vi "Three part faster.vi"() -> ()   [LabVIEW 2009]
uses:
  <vilib>/vision/Image Controls.llb/IMAQ Image.ctl
  <vilib>/Analysis/3filter.llb/Filter Passband Type.ctl
  <vilib>/Analysis/3filter.llb/Butterworth Filter (DBL).vi
  <vilib>/Instr/_visa.llb/VISA Configure Serial Port (Instr).vi
  <vilib>/vision/NI_Vision_Development_Module.lvlib
  <vilib>/Analysis/NI_AALBase.lvlib
panel:
  out "decimal integer string 2":string
  out "number 2":u32
  out "cluster 2":T1
  in  "Orange Guitar":T2={"Global Rectangle"=[587, 282, 628, 378], "Contours"=[{"ID"=enum."External", "Type"=2, "Coordinates"=[627, 377, 587, 282]}]} {"Contours"."Type" items=["No Selection", "Point", "Line", "Rectangle", "Oval", "Polygon", "Freehand Region", "Annulus", "Unused2", "Unused3", "Broken Line", "Freehand Line", "Rotated Rectangle"]}
  in  "Yellow Guitar":T2={"Global Rectangle"=[546, 282, 563, 376], "Contours"=[{"ID"=enum."External", "Type"=2, "Coordinates"=[562, 375, 546, 282]}]} {"Contours"."Type" items=["No Selection", "Point", "Line", "Rectangle", "Oval", "Polygon", "Freehand Region", "Annulus", "Unused2", "Unused3", "Broken Line", "Freehand Line", "Rotated Rectangle"]}
  in  "Green Guitar":T2={"Global Rectangle"=[498, 284, 505, 376], "Contours"=[{"ID"=enum."External", "Type"=2, "Coordinates"=[498, 375, 504, 284]}]} {"Contours"."Type" items=["No Selection", "Point", "Line", "Rectangle", "Oval", "Polygon", "Freehand Region", "Annulus", "Unused2", "Unused3", "Broken Line", "Freehand Line", "Rotated Rectangle"]}
  in  "Blue Guitar":T2={"Global Rectangle"=[569, 290, 594, 372], "Contours"=[{"ID"=enum."External", "Type"=2, "Coordinates"=[593, 371, 569, 290]}]} {"Contours"."Type" items=["No Selection", "Point", "Line", "Rectangle", "Oval", "Polygon", "Freehand Region", "Annulus", "Unused2", "Unused3", "Broken Line", "Freehand Line", "Rotated Rectangle"]}
  in  "Red Guitar":T2={"Global Rectangle"=[526, 284, 530, 370], "Contours"=[{"ID"=enum."External", "Type"=2, "Coordinates"=[529, 369, 526, 284]}]} {"Contours"."Type" items=["No Selection", "Point", "Line", "Rectangle", "Oval", "Polygon", "Freehand Region", "Annulus", "Unused2", "Unused3", "Broken Line", "Freehand Line", "Rotated Rectangle"]}
  out "Blue Guitar":dbl[](graph)
  out "Yellow Guitar":dbl[](graph)
  out "Yellow Guitar LED":bool
  out "Green Guitar":dbl[](graph)
  out "Green Guitar LED":bool
  out "Red Guitar":dbl[](graph)
  out "Red Guitar LED":bool
  out "Blue Guitar LED":bool
  out "Orange Guitar":dbl[](graph)
  out "Orange Guitar LED":bool
  in  "Orange Bass":T2={"Global Rectangle"=[220, 296, 225, 371], "Contours"=[{"ID"=enum."External", "Type"=2, "Coordinates"=[224, 370, 220, 296]}]} {"Contours"."Type" items=["No Selection", "Point", "Line", "Rectangle", "Oval", "Polygon", "Freehand Region", "Annulus", "Unused2", "Unused3", "Broken Line", "Freehand Line", "Rotated Rectangle"]}
  out "Orange Bass":dbl[](graph)
  out "Orange Bass LED":bool
  in  "Green Bass":T2={"Global Rectangle"=[100, 292, 131, 371], "Contours"=[{"ID"=enum."External", "Type"=2, "Coordinates"=[100, 370, 130, 292]}]} {"Contours"."Type" items=["No Selection", "Point", "Line", "Rectangle", "Oval", "Polygon", "Freehand Region", "Annulus", "Unused2", "Unused3", "Broken Line", "Freehand Line", "Rotated Rectangle"]}
  in  "Blue Bass":T2={"Global Rectangle"=[193, 293, 199, 374], "Contours"=[{"ID"=enum."External", "Type"=2, "Coordinates"=[193, 373, 198, 293]}]} {"Contours"."Type" items=["No Selection", "Point", "Line", "Rectangle", "Oval", "Polygon", "Freehand Region", "Annulus", "Unused2", "Unused3", "Broken Line", "Freehand Line", "Rotated Rectangle"]}
  in  "Red Bass":T2={"Global Rectangle"=[129, 294, 154, 376], "Contours"=[{"ID"=enum."External", "Type"=2, "Coordinates"=[129, 375, 153, 294]}]} {"Contours"."Type" items=["No Selection", "Point", "Line", "Rectangle", "Oval", "Polygon", "Freehand Region", "Annulus", "Unused2", "Unused3", "Broken Line", "Freehand Line", "Rotated Rectangle"]}
  in  "Yellow Bass":T2={"Global Rectangle"=[160, 295, 175, 378], "Contours"=[{"ID"=enum."External", "Type"=2, "Coordinates"=[160, 377, 174, 295]}]} {"Contours"."Type" items=["No Selection", "Point", "Line", "Rectangle", "Oval", "Polygon", "Freehand Region", "Annulus", "Unused2", "Unused3", "Broken Line", "Freehand Line", "Rotated Rectangle"]}
  out "Blue Bass":dbl[](graph)
  out "Yellow Bass":dbl[](graph)
  out "Yellow Bass LED":bool
  out "Green Bass":dbl[](graph)
  out "Green Bass LED":bool
  out "Red Bass":dbl[](graph)
  out "Red Bass LED":bool
  out "Blue Bass LED":bool
  in  "Mask":T2 {"Contours"."Type" items=["No Selection", "Point", "Line", "Rectangle", "Oval", "Polygon", "Freehand Region", "Annulus", "Unused2", "Unused3", "Broken Line", "Freehand Line", "Rotated Rectangle"]}
  in  "Red Line":T2={"Global Rectangle"=[300, 297, 320, 380], "Contours"=[{"ID"=enum."External", "Type"=2, "Coordinates"=[300, 379, 319, 297]}]} {"Contours"."Type" items=["No Selection", "Point", "Line", "Rectangle", "Oval", "Polygon", "Freehand Region", "Annulus", "Unused2", "Unused3", "Broken Line", "Freehand Line", "Rotated Rectangle"]}
  out "Waveform Red":dbl[](graph)
  out "LED Red":bool
  in  "Blue Line":T2={"Global Rectangle"=[374, 278, 383, 377], "Contours"=[{"ID"=enum."External", "Type"=2, "Coordinates"=[382, 376, 374, 278]}]} {"Contours"."Type" items=["No Selection", "Point", "Line", "Rectangle", "Oval", "Polygon", "Freehand Region", "Annulus", "Unused2", "Unused3", "Broken Line", "Freehand Line", "Rotated Rectangle"]}
  in  "Green Line":T2={"Global Rectangle"=[406, 309, 423, 383], "Contours"=[{"ID"=enum."External", "Type"=2, "Coordinates"=[422, 382, 406, 309]}]} {"Contours"."Type" items=["No Selection", "Point", "Line", "Rectangle", "Oval", "Polygon", "Freehand Region", "Annulus", "Unused2", "Unused3", "Broken Line", "Freehand Line", "Rotated Rectangle"]}
  out "Waveform Green":dbl[](graph)
  out "LED Green":bool
  in  "Yellow Line":T2={"Global Rectangle"=[342, 292, 349, 377], "Contours"=[{"ID"=enum."External", "Type"=2, "Coordinates"=[342, 376, 348, 292]}]} {"Contours"."Type" items=["No Selection", "Point", "Line", "Rectangle", "Oval", "Polygon", "Freehand Region", "Annulus", "Unused2", "Unused3", "Broken Line", "Freehand Line", "Rotated Rectangle"]}
  out "cluster":T1
  in  "baud rate (9600)":u32=9600
  in  "VISA resource name":refnum<visa-resource-name>
  out "number":u32
  out "decimal integer string":string
  out "Image Dst Out":T3
  out "LED Yellow":bool
  out "Waveform Yellow":dbl[](graph)
  in  "playtime":dbl=30.0
  out "Frame Number":i32
  in  "Frame Start":i32=2400
  out "Blue Drum":bool
  out "Blue Drum":dbl[](graph)
  in  "stop":bool
  in  "AVI Path":path
  # "BLUE"
  # "YELLOW"
  # "GREEN"
  # "RED"
  # "Drums"
  # "Bass"
  # "Guitar"
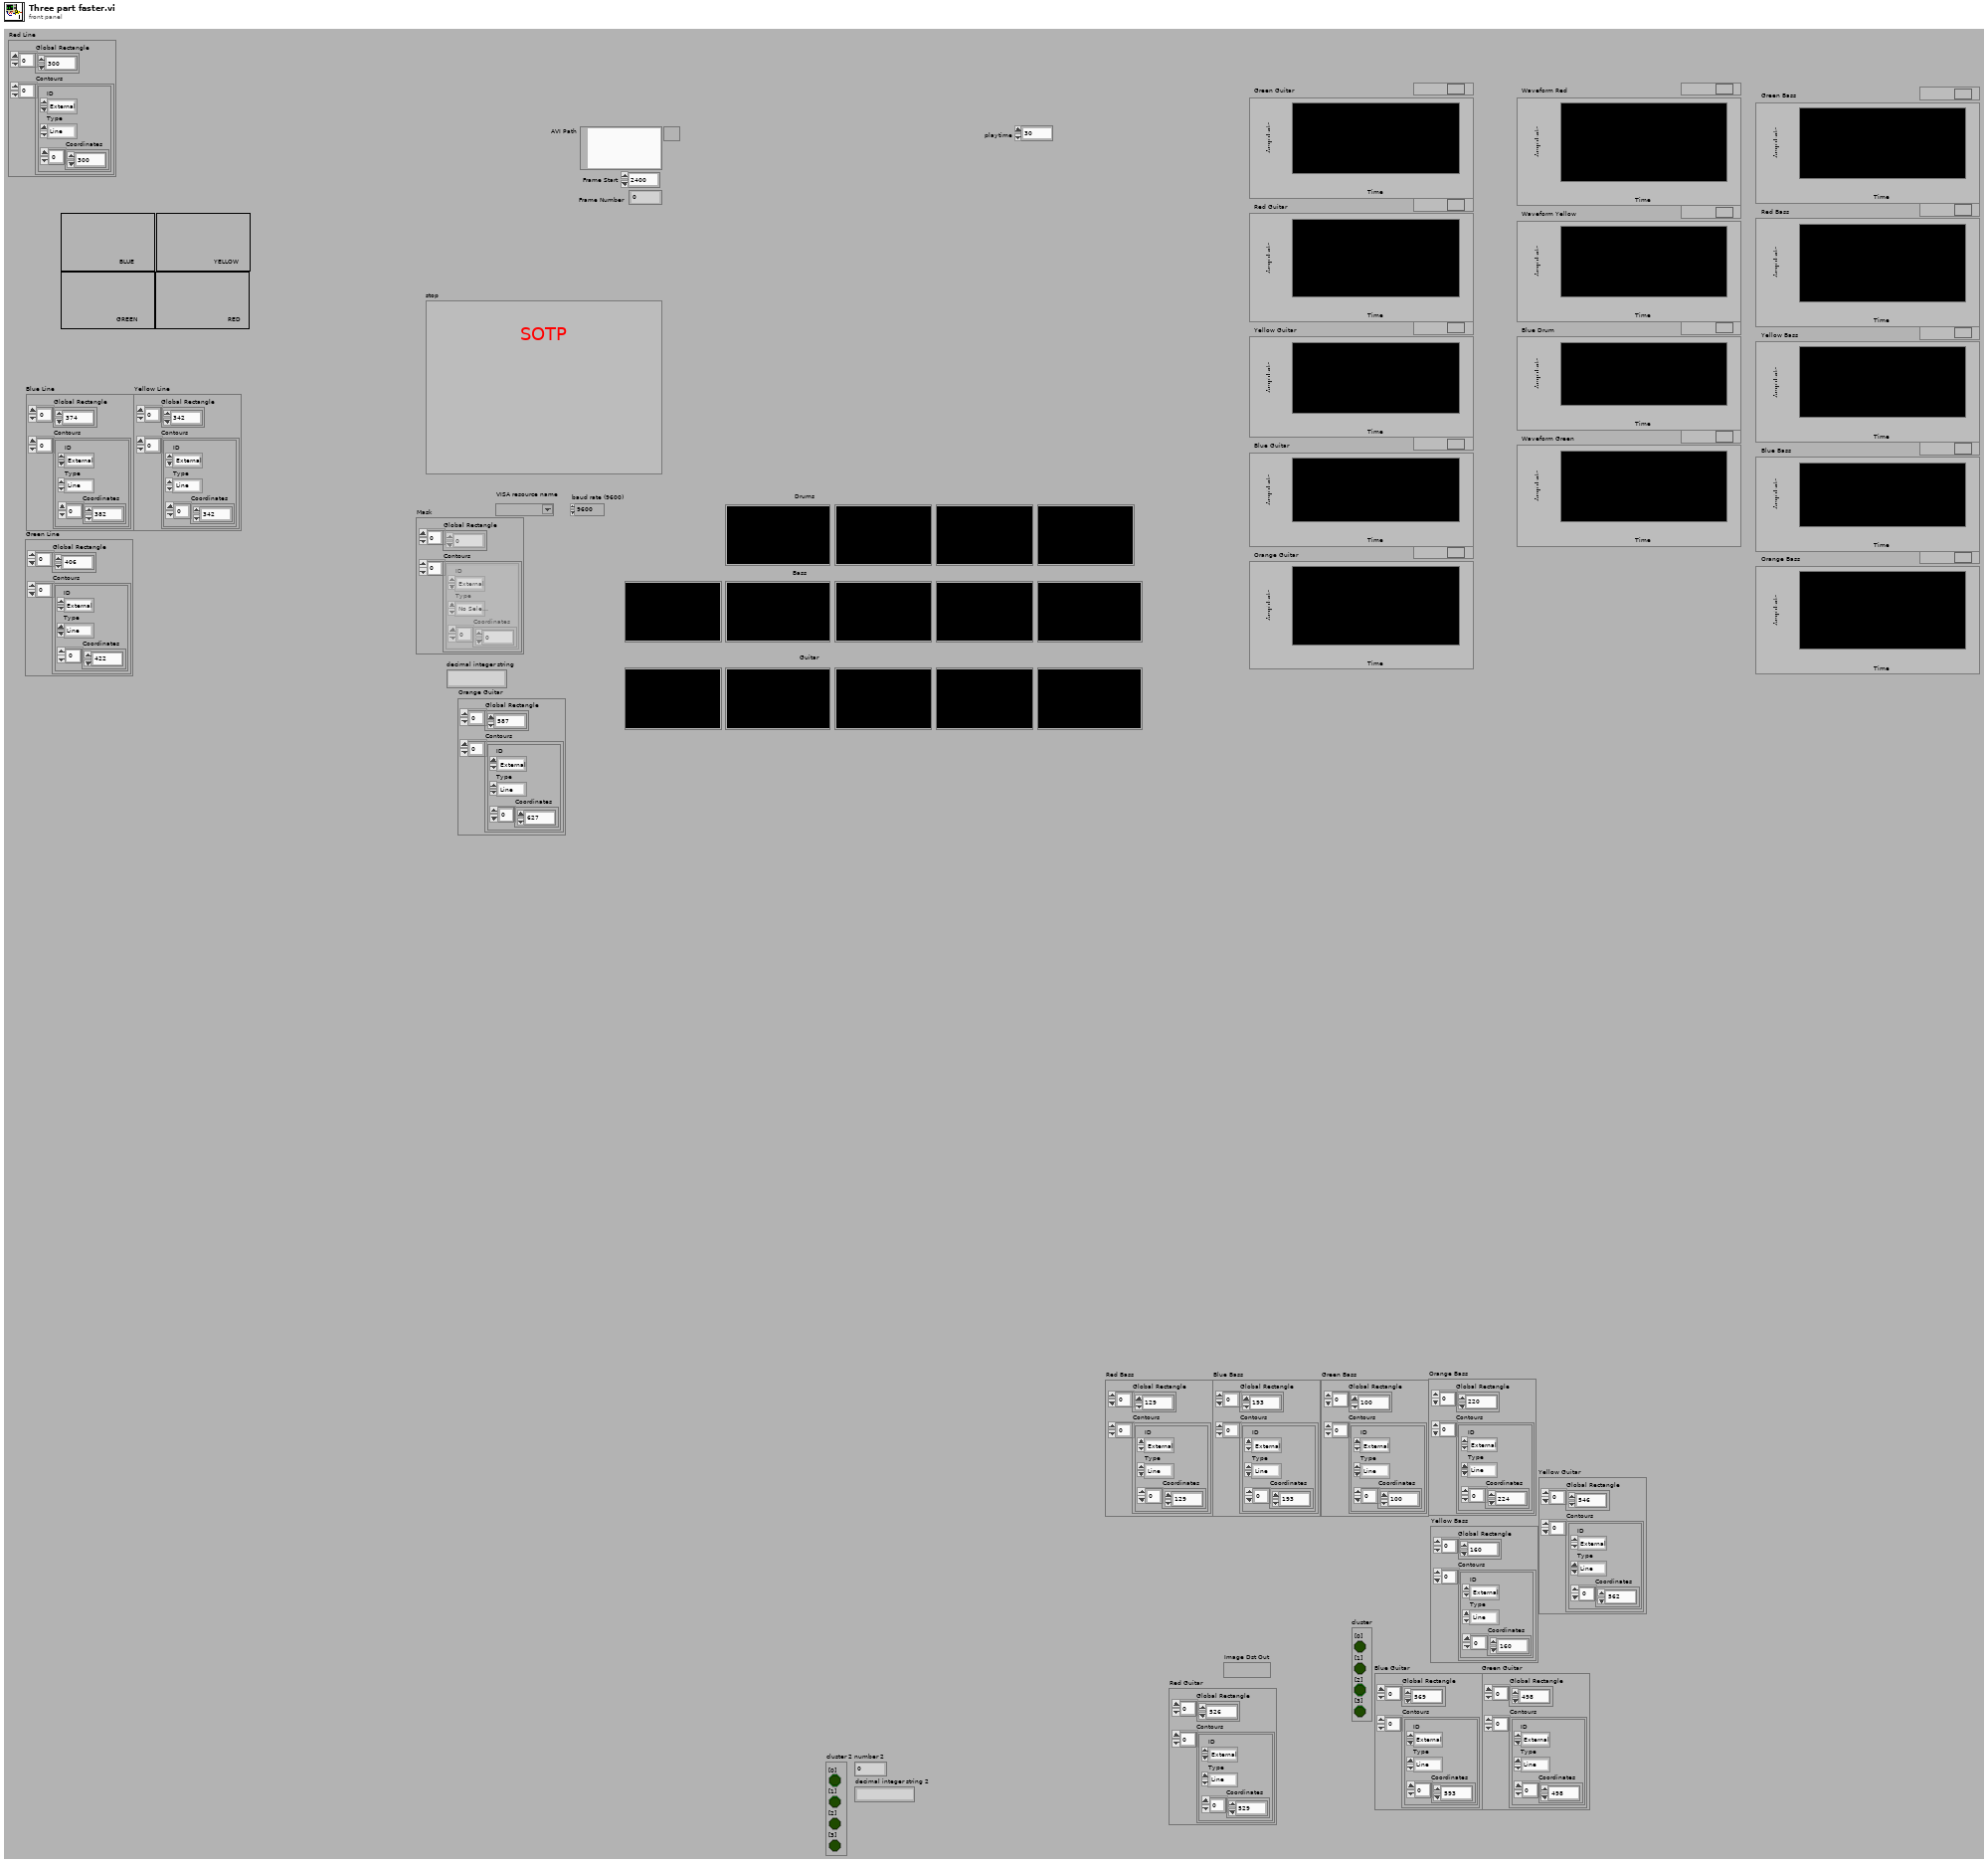
[diagram p1: front panel]
types:
  T1 = cluster{"[0]":bool, "[1]":bool, "[2]":bool, "[3]":bool, "[4]":bool, "[5]":bool, "[6]":bool, "[7]":bool, "[8]":bool}
  T2 = cluster{"Global Rectangle":i32[], "Contours":cluster{"ID":enum32{"External", "Internal"}, "Type":u32, "Coordinates":i32[]}[]}
  T3 = typedef "IMAQ Image.ctl" = refnum<image>
  T4 = typedef "NI_AALBase.lvlib/Filter Passband Type.ctl" = enum32{"Lowpass", "Highpass", "Bandpass", "Bandstop"}
  T5 = typedef "Image Type" = u32
  T6 = typedef "AviRefnum.ctl" = refnum<k1>
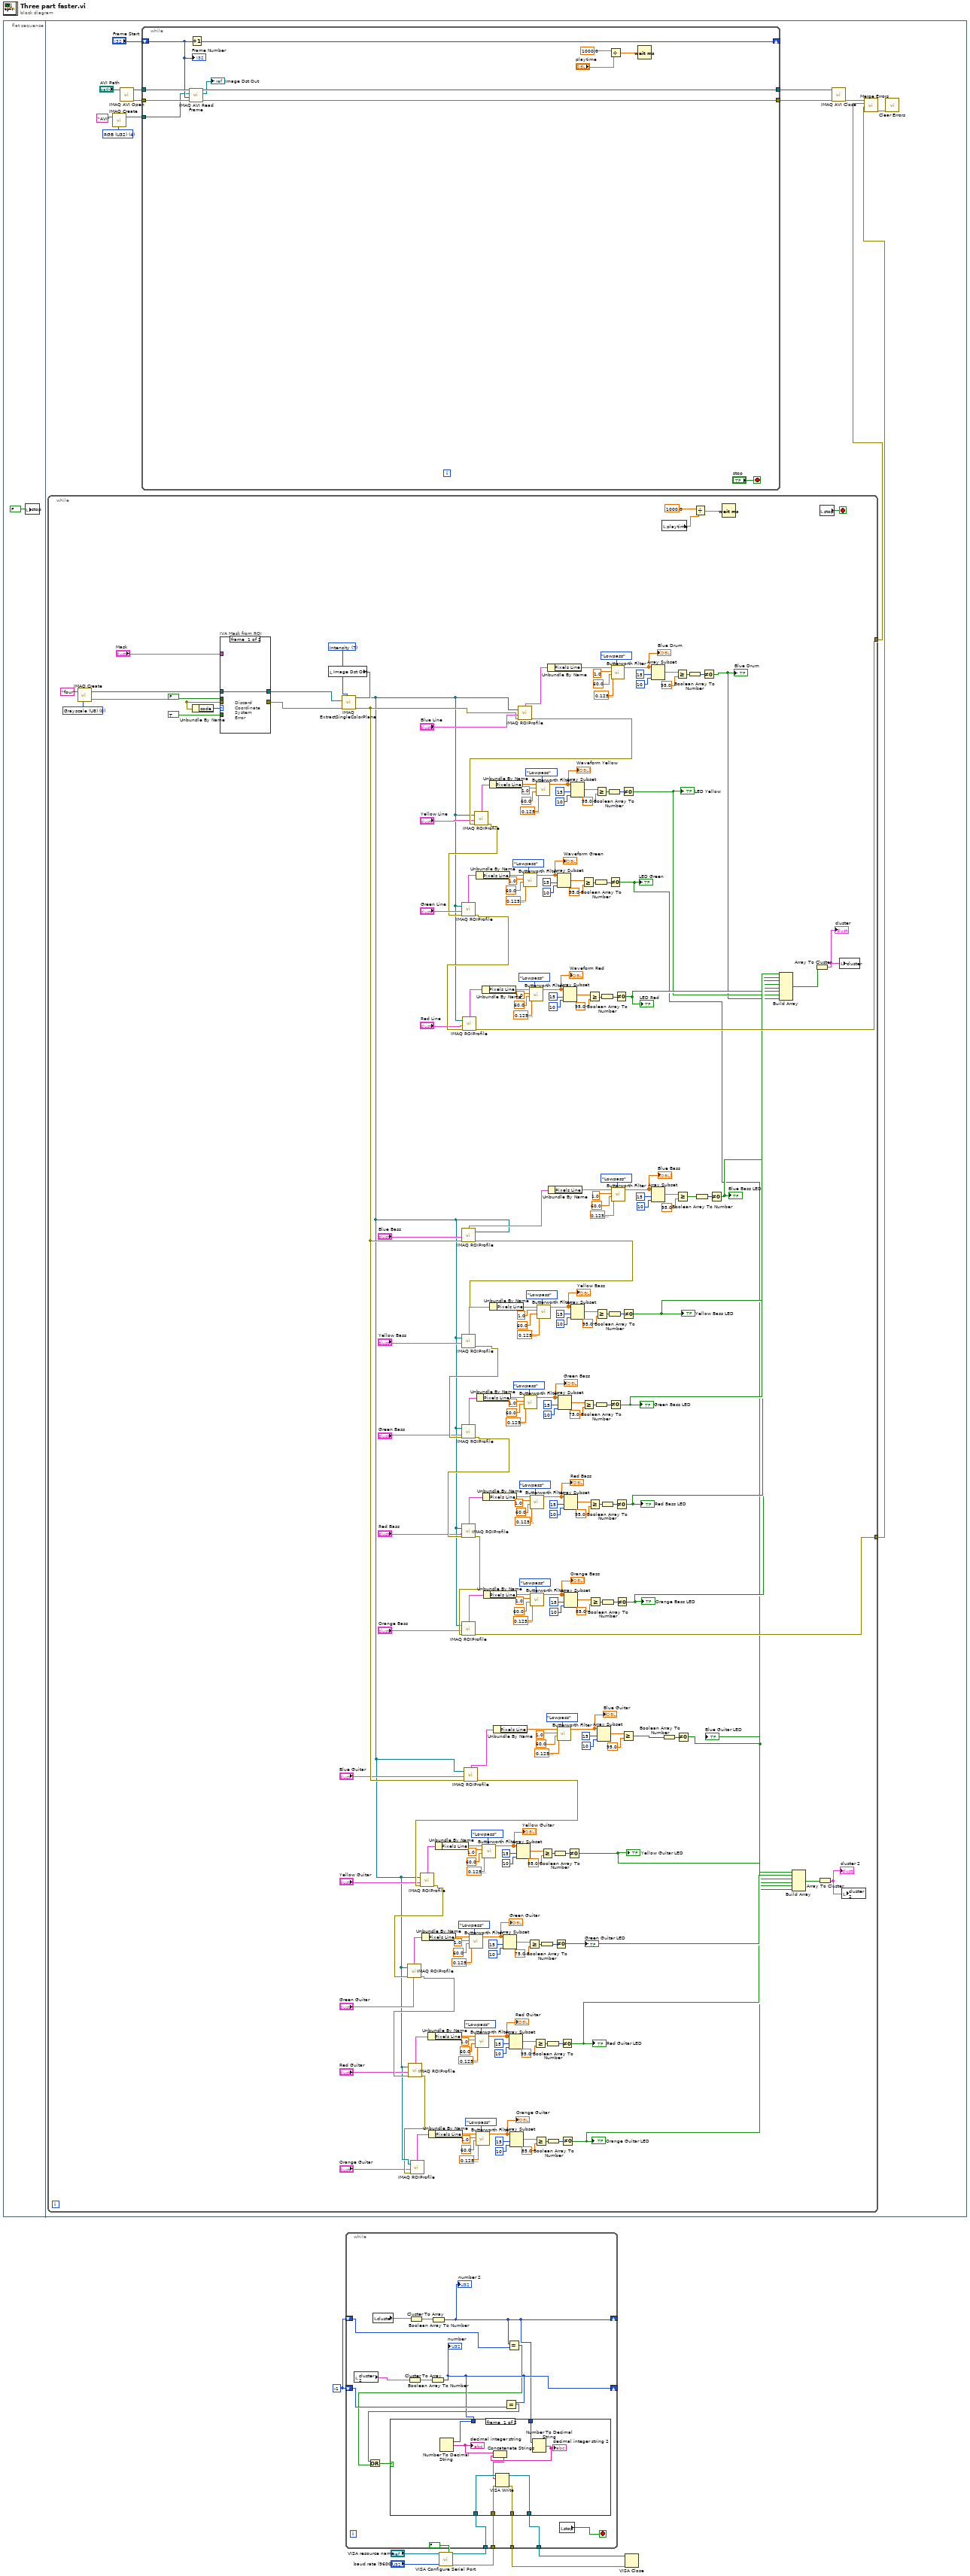
[diagram p0: block diagram]
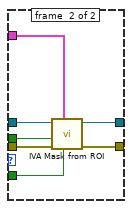
[diagram p3: hidden frame]
diagram:
  w1 = -1
  n1 = flat-sequence {
    frame #0 {
      n2 = local write "stop"(FALSE ("stop")) -> ()
    }
    frame #1 {
      w14 = T5 4 items=["Grayscale (U8)", "Grayscale (I16)", "Grayscale (SGL)", "Complex (CSG)", "RGB (U32)", "HSL (U32)", "RGB (U64)", "Grayscale (U16)"] ("Image Type")
      n3 = while {
        tunnel: [w251] -> w11
        tunnel: [w117] -> w10
        stop <- w266 stop-if-true
        w261 = T5 0 items=["Grayscale (U8)", "Grayscale (I16)", "Grayscale (SGL)", "Complex (CSG)", "RGB (U32)", "HSL (U32)", "RGB (U64)", "Grayscale (U16)"] ("Image Type")
        w267 = 7 items=["Red", "Green", "Blue", "Hue", "Saturation", "Luminance", "Value", "Intensity"] ("Color Plane")
        n4 = call "IMAQ Create"("Image Name"="four", "Image Type"=w261) -> ("New Image"=w254:T3, "error out"=w255:errorcluster)  [unwired: 3 in]
        n5 = Unbundle By Name(w255) -> ("code"=w259:i32)
        n6 = case "IVA Mask from ROI" shown="Default" w259 {
          tunnel: "Mask" -> [_ w275]
          tunnel: TRUE ("Shrink") -> [_ w274]
          tunnel: w254 -> [w268 w273]
          tunnel: w255 -> [_ w272]
          tunnel: [_ w271] -> w256
          tunnel: [w268 w270] -> w252
          tunnel: FALSE ("Out / In") -> [_ w269]
          frame #0 {
            # "Discard\nCoordinate\nSystem\nError"
          }
          frame #1 {
            n7 = call <vilib>:"IVA Mask from ROI.vi"("Shrink"=w274, "ROI Descriptor"=w275, "error in (no error)"=w272, "Out / In"=w269, "Image Src"=w273) -> ("error out"=w271:errorcluster, "Image Out"=w270:T3)  [unwired: 5 out]
          }
        }
        n8 = local read "Image Dst Out"() -> (w262:T3)
        n9 = call "IMAQ ExtractSingleColorPlane"("Color Plane"=w267, "error in (no error)"=w256, "Image Dst"=w252, "Image Src"=w262) -> ("error out"=w39:errorcluster, "Image Dst Out"=w34:T3)  [unwired: 6 out]
        n10 = call "IMAQ ROIProfile"("error in (no error)"=w39, "ROI Descriptor"="Blue Bass", "Image"=w34) -> ("error out"=w166:errorcluster, "ROI Graph"=w165:cluster{"x0":sgl, "dx":sgl, "Pixels Line":sgl[]})  [unwired: 4 out]
        n11 = call "IMAQ ROIProfile"("error in (no error)"=w166, "ROI Descriptor"="Yellow Bass", "Image"=w34) -> ("error out"=w136:errorcluster, "ROI Graph"=w169:cluster{"x0":sgl, "dx":sgl, "Pixels Line":sgl[]})  [unwired: 4 out]
        n12 = call "IMAQ ROIProfile"("error in (no error)"=w136, "ROI Descriptor"="Green Bass", "Image"=w34) -> ("error out"=w137:errorcluster, "ROI Graph"=w163:cluster{"x0":sgl, "dx":sgl, "Pixels Line":sgl[]})  [unwired: 4 out]
        n13 = call "IMAQ ROIProfile"("error in (no error)"=w137, "ROI Descriptor"="Red Bass", "Image"=w34) -> ("error out"=w118:errorcluster, "ROI Graph"=w139:cluster{"x0":sgl, "dx":sgl, "Pixels Line":sgl[]})  [unwired: 4 out]
        n14 = call "IMAQ ROIProfile"("error in (no error)"=w118, "ROI Descriptor"="Orange Bass", "Image"=w34) -> ("error out"=w117:errorcluster, "ROI Graph"=w130:cluster{"x0":sgl, "dx":sgl, "Pixels Line":sgl[]})  [unwired: 4 out]
        n15 = call "IMAQ ROIProfile"("error in (no error)"=w39, "ROI Descriptor"="Blue Guitar", "Image"=w34) -> ("error out"=w63:errorcluster, "ROI Graph"=w64:cluster{"x0":sgl, "dx":sgl, "Pixels Line":sgl[]})  [unwired: 4 out]
        n16 = call "IMAQ ROIProfile"("error in (no error)"=w63, "ROI Descriptor"="Yellow Guitar", "Image"=w34) -> ("error out"=w93:errorcluster, "ROI Graph"=w60:cluster{"x0":sgl, "dx":sgl, "Pixels Line":sgl[]})  [unwired: 4 out]
        n17 = call "IMAQ ROIProfile"("error in (no error)"=w93, "ROI Descriptor"="Green Guitar", "Image"=w34) -> ("error out"=w92:errorcluster, "ROI Graph"=w66:cluster{"x0":sgl, "dx":sgl, "Pixels Line":sgl[]})  [unwired: 4 out]
        n18 = call "IMAQ ROIProfile"("error in (no error)"=w92, "ROI Descriptor"="Red Guitar", "Image"=w34) -> ("error out"=w33:errorcluster, "ROI Graph"=w90:cluster{"x0":sgl, "dx":sgl, "Pixels Line":sgl[]})  [unwired: 4 out]
        n19 = call "IMAQ ROIProfile"("error in (no error)"=w33, "ROI Descriptor"="Orange Guitar", "Image"=w34) -> ("ROI Graph"=w32:cluster{"x0":sgl, "dx":sgl, "Pixels Line":sgl[]})  [unwired: 5 out]
        n20 = Unbundle By Name(w66) -> ("Pixels Line"=w69:sgl[])
        n21 = Unbundle By Name(w90) -> ("Pixels Line"=w87:sgl[])
        n22 = Unbundle By Name(w32) -> ("Pixels Line"=w97:sgl[])
        n23 = Unbundle By Name(w60) -> ("Pixels Line"=w57:sgl[])
        n24 = call-poly <vilib>:"Butterworth Filter.vi"("filter type"=Filter_Passband_Type."Lowpass", "low cutoff freq: fl"=0.12500000000000006 ("low  11"), "high cutoff freq: fh"=60.0 ("high 12"), "sampling freq: fs"=1.0 ("sampling 11"), "X"=w69) -> ("Filtered X"=w65:dbl[])  [unwired: 3 in, 1 out]
        "Green Guitar" <- w65
        n25 = call-poly <vilib>:"Butterworth Filter.vi"("filter type"=Filter_Passband_Type."Lowpass", "low cutoff freq: fl"=0.12500000000000006 ("low  10"), "high cutoff freq: fh"=60.0 ("high 11"), "sampling freq: fs"=1.0 ("sampling 10"), "X"=w87) -> ("Filtered X"=w91:dbl[])  [unwired: 3 in, 1 out]
        "Red Guitar" <- w91
        n26 = call-poly <vilib>:"Butterworth Filter.vi"("filter type"=Filter_Passband_Type."Lowpass", "low cutoff freq: fl"=0.12500000000000006 ("low  9"), "high cutoff freq: fh"=60.0 ("high 10"), "sampling freq: fs"=1.0 ("sampling 9"), "X"=w97) -> ("Filtered X"=w94:dbl[])  [unwired: 3 in, 1 out]
        "Orange Guitar" <- w94
        n27 = Unbundle By Name(w163) -> ("Pixels Line"=w160:sgl[])
        n28 = call-poly <vilib>:"Butterworth Filter.vi"("filter type"=Filter_Passband_Type."Lowpass", "low cutoff freq: fl"=0.12500000000000006 ("low  12"), "high cutoff freq: fh"=60.0 ("high 13"), "sampling freq: fs"=1.0 ("sampling 12"), "X"=w57) -> ("Filtered X"=w61:dbl[])  [unwired: 3 in, 1 out]
        "Yellow Guitar" <- w61
        n29 = Unbundle By Name(w139) -> ("Pixels Line"=w142:sgl[])
        n30 = Unbundle By Name(w130) -> ("Pixels Line"=w127:sgl[])
        n31 = Unbundle By Name(w169) -> ("Pixels Line"=w172:sgl[])
        n32 = Unbundle By Name(w64) -> ("Pixels Line"=w41:sgl[])
        n33 = Array Subset(array=w65, index=15, length=10) -> (w74:dbl[])
        n34 = Array Subset(array=w91, index=15, length=10) -> (w82:dbl[])
        n35 = Array Subset(array=w94, index=15, length=10) -> (w102:dbl[])
        n36 = Array Subset(array=w61, index=15, length=10) -> (w52:dbl[])
        n37 = call "IMAQ ROIProfile"("error in (no error)"=w39, "ROI Descriptor"="Blue Line", "Image"=w34) -> ("error out"=w226:errorcluster, "ROI Graph"=w225:cluster{"x0":sgl, "dx":sgl, "Pixels Line":sgl[]})  [unwired: 4 out]
        n38 = call "IMAQ ROIProfile"("error in (no error)"=w226, "ROI Descriptor"="Yellow Line", "Image"=w34) -> ("error out"=w193:errorcluster, "ROI Graph"=w229:cluster{"x0":sgl, "dx":sgl, "Pixels Line":sgl[]})  [unwired: 4 out]
        n39 = call "IMAQ ROIProfile"("error in (no error)"=w193, "ROI Descriptor"="Green Line", "Image"=w34) -> ("error out"=w196:errorcluster, "ROI Graph"=w223:cluster{"x0":sgl, "dx":sgl, "Pixels Line":sgl[]})  [unwired: 4 out]
        n40 = call "IMAQ ROIProfile"("error in (no error)"=w196, "ROI Descriptor"="Red Line", "Image"=w34) -> ("error out"=w251:errorcluster, "ROI Graph"=w198:cluster{"x0":sgl, "dx":sgl, "Pixels Line":sgl[]})  [unwired: 4 out]
        n41 = Unbundle By Name(w223) -> ("Pixels Line"=w220:sgl[])
        n42 = Unbundle By Name(w198) -> ("Pixels Line"=w201:sgl[])
        n43 = Unbundle By Name(w229) -> ("Pixels Line"=w232:sgl[])
        n44 = call-poly <vilib>:"Butterworth Filter.vi"("filter type"=Filter_Passband_Type."Lowpass", "low cutoff freq: fl"=0.12500000000000006 ("low  3"), "high cutoff freq: fh"=60.0 ("high 3"), "sampling freq: fs"=1.0 ("sampling 3"), "X"=w220) -> ("Filtered X"=w224:dbl[])  [unwired: 3 in, 1 out]
        "Waveform Green" <- w224
        n45 = call-poly <vilib>:"Butterworth Filter.vi"("filter type"=Filter_Passband_Type."Lowpass", "low cutoff freq: fl"=0.12500000000000006 ("low  6"), "high cutoff freq: fh"=60.0 ("high 6"), "sampling freq: fs"=1.0 ("sampling 6"), "X"=w160) -> ("Filtered X"=w164:dbl[])  [unwired: 3 in, 1 out]
        "Green Bass" <- w164
        n46 = Greater Or Equal?(x=w74, y=75.0) -> (x >= y?=w72:bool[])
        n47 = call-poly <vilib>:"Butterworth Filter.vi"("filter type"=Filter_Passband_Type."Lowpass", "low cutoff freq: fl"=0.12500000000000006 ("low  4"), "high cutoff freq: fh"=60.0 ("high 4"), "sampling freq: fs"=1.0 ("sampling 4"), "X"=w201) -> ("Filtered X"=w197:dbl[])  [unwired: 3 in, 1 out]
        "Waveform Red" <- w197
        n48 = call-poly <vilib>:"Butterworth Filter.vi"("filter type"=Filter_Passband_Type."Lowpass", "low cutoff freq: fl"=0.12500000000000006 ("low  5"), "high cutoff freq: fh"=60.0 ("high 5"), "sampling freq: fs"=1.0 ("sampling 5"), "X"=w142) -> ("Filtered X"=w138:dbl[])  [unwired: 3 in, 1 out]
        "Red Bass" <- w138
        n49 = call-poly <vilib>:"Butterworth Filter.vi"("filter type"=Filter_Passband_Type."Lowpass", "low cutoff freq: fl"=0.12500000000000006 ("low  8"), "high cutoff freq: fh"=60.0 ("high 9"), "sampling freq: fs"=1.0 ("sampling 8"), "X"=w127) -> ("Filtered X"=w131:dbl[])  [unwired: 3 in, 1 out]
        "Orange Bass" <- w131
        n50 = Greater Or Equal?(x=w82, y=95.0) -> (x >= y?=w84:bool[])
        n51 = Greater Or Equal?(x=w102, y=85.0) -> (x >= y?=w100:bool[])
        n52 = call-poly <vilib>:"Butterworth Filter.vi"("filter type"=Filter_Passband_Type."Lowpass", "low cutoff freq: fl"=0.12500000000000006 ("low  2"), "high cutoff freq: fh"=60.0 ("high 2"), "sampling freq: fs"=1.0 ("sampling 2"), "X"=w232) -> ("Filtered X"=w228:dbl[])  [unwired: 3 in, 1 out]
        "Waveform Yellow" <- w228
        n53 = call-poly <vilib>:"Butterworth Filter.vi"("filter type"=Filter_Passband_Type."Lowpass", "low cutoff freq: fl"=0.12500000000000006 ("low  7"), "high cutoff freq: fh"=60.0 ("high 7"), "sampling freq: fs"=1.0 ("sampling 7"), "X"=w172) -> ("Filtered X"=w168:dbl[])  [unwired: 3 in, 1 out]
        "Yellow Bass" <- w168
        n54 = Boolean Array To Number(Boolean array=w72) -> (number=w71:u32)
        n55 = Greater Or Equal?(x=w52, y=95.0) -> (x >= y?=w54:bool[])
        n56 = Boolean Array To Number(Boolean array=w84) -> (number=w85:u32)
        n57 = Boolean Array To Number(Boolean array=w100) -> (number=w99:u32)
        n58 = Unbundle By Name(w225) -> ("Pixels Line"=w249:sgl[])
        n59 = Unbundle By Name(w165) -> ("Pixels Line"=w188:sgl[])
        n60 = Boolean Array To Number(Boolean array=w54) -> (number=w55:u32)
        n61 = Not Equal To 0?(x=w71) -> (x != 0?=w29:bool)
        "Green Guitar LED" <- w29
        n62 = call-poly <vilib>:"Butterworth Filter.vi"("filter type"=Filter_Passband_Type."Lowpass", "low cutoff freq: fl"=0.12500000000000006 ("low 3"), "high cutoff freq: fh"=60.0 ("high 14"), "sampling freq: fs"=1.0 ("sampling  9"), "X"=w41) -> ("Filtered X"=w78:dbl[])  [unwired: 3 in, 1 out]
        "Blue Guitar" <- w78
        n63 = Array Subset(array=w224, index=15, length=10) -> (w215:dbl[])
        n64 = Array Subset(array=w164, index=15, length=10) -> (w155:dbl[])
        n65 = Not Equal To 0?(x=w85) -> (x != 0?=w28:bool)
        "Red Guitar LED" <- w28
        n66 = Not Equal To 0?(x=w99) -> (x != 0?=w25:bool)
        "Orange Guitar LED" <- w25
        n67 = Array Subset(array=w197, index=15, length=10) -> (w206:dbl[])
        n68 = Array Subset(array=w138, index=15, length=10) -> (w147:dbl[])
        n69 = Array Subset(array=w131, index=15, length=10) -> (w122:dbl[])
        n70 = Not Equal To 0?(x=w55) -> (x != 0?=w27:bool)
        "Yellow Guitar LED" <- w27
        n71 = Array Subset(array=w228, index=15, length=10) -> (w237:dbl[])
        n72 = Array Subset(array=w168, index=15, length=10) -> (w177:dbl[])
        n73 = Greater Or Equal?(x=w215, y=95.0) -> (x >= y?=w217:bool[])
        n74 = Greater Or Equal?(x=w155, y=75.0) -> (x >= y?=w157:bool[])
        n75 = Greater Or Equal?(x=w206, y=95.0) -> (x >= y?=w204:bool[])
        n76 = Greater Or Equal?(x=w147, y=95.0) -> (x >= y?=w145:bool[])
        n77 = Greater Or Equal?(x=w122, y=85.0) -> (x >= y?=w124:bool[])
        n78 = Boolean Array To Number(Boolean array=w217) -> (number=w218:u32)
        n79 = Greater Or Equal?(x=w237, y=95.0) -> (x >= y?=w235:bool[])
        n80 = Boolean Array To Number(Boolean array=w157) -> (number=w158:u32)
        n81 = Greater Or Equal?(x=w177, y=95.0) -> (x >= y?=w175:bool[])
        n82 = Array Subset(array=w78, index=15, length=10) -> (w47:dbl[])
        n83 = Boolean Array To Number(Boolean array=w204) -> (number=w203:u32)
        n84 = Boolean Array To Number(Boolean array=w145) -> (number=w144:u32)
        n85 = Boolean Array To Number(Boolean array=w124) -> (number=w125:u32)
        n86 = Boolean Array To Number(Boolean array=w235) -> (number=w234:u32)
        n87 = Boolean Array To Number(Boolean array=w175) -> (number=w174:u32)
        n88 = Not Equal To 0?(x=w218) -> (x != 0?=w30:bool)
        "LED Green" <- w30
        n89 = Not Equal To 0?(x=w158) -> (x != 0?=w115:bool)
        "Green Bass LED" <- w115
        n90 = call-poly <vilib>:"Butterworth Filter.vi"("filter type"=Filter_Passband_Type."Lowpass", "low cutoff freq: fl"=0.12500000000000006 ("low"), "high cutoff freq: fh"=60.0 ("high"), "sampling freq: fs"=1.0 ("sampling"), "X"=w249) -> ("Filtered X"=w211:dbl[])  [unwired: 3 in, 1 out]
        "Blue Drum" <- w211
        n91 = call-poly <vilib>:"Butterworth Filter.vi"("filter type"=Filter_Passband_Type."Lowpass", "low cutoff freq: fl"=0.12500000000000006 ("low 2"), "high cutoff freq: fh"=60.0 ("high 8"), "sampling freq: fs"=1.0 ("sampling  8"), "X"=w188) -> ("Filtered X"=w151:dbl[])  [unwired: 3 in, 1 out]
        "Blue Bass" <- w151
        n92 = Not Equal To 0?(x=w203) -> (x != 0?=w110:bool)
        "LED Red" <- w110
        n93 = Not Equal To 0?(x=w144) -> (x != 0?=w114:bool)
        "Red Bass LED" <- w114
        n94 = Not Equal To 0?(x=w125) -> (x != 0?=w111:bool)
        "Orange Bass LED" <- w111
        n95 = Not Equal To 0?(x=w234) -> (x != 0?=w109:bool)
        "LED Yellow" <- w109
        n96 = Greater Or Equal?(x=w47, y=95.0) -> (x >= y?=w106:bool[])
        n97 = Not Equal To 0?(x=w174) -> (x != 0?=w113:bool)
        "Yellow Bass LED" <- w113
        n98 = Array Subset(array=w211, index=15, length=10) -> (w243:dbl[])
        n99 = Array Subset(array=w151, index=15, length=10) -> (w182:dbl[])
        n100 = local read "playtime"() -> (w263:dbl)
        n101 = Boolean Array To Number(Boolean array=w106) -> (number=w49:u32)
        n102 = Greater Or Equal?(x=w243, y=95.0) -> (x >= y?=w241:bool[])
        n103 = Greater Or Equal?(x=w182, y=95.0) -> (x >= y?=w107:bool[])
        n104 = Not Equal To 0?(x=w49) -> (x != 0?=w26:bool)
        "Blue Guitar LED" <- w26
        n105 = Boolean Array To Number(Boolean array=w241) -> (number=w240:u32)
        n106 = Divide(x=1000.0, y=w263) -> (x/y=w265:dbl)
        n107 = Boolean Array To Number(Boolean array=w107) -> (number=w180:u32)
        n108 = Not Equal To 0?(x=w240) -> (x != 0?=w108:bool)
        "Blue Drum" <- w108
        n109 = Not Equal To 0?(x=w180) -> (x != 0?=w112:bool)
        "Blue Bass LED" <- w112
        n110 = Wait (ms)(milliseconds to wait=w265) -> ()  [unwired: 1 out]
        n111 = Build Array(w115, w114, w113, w112, w111, w110, w109, w108) -> (w191:bool[])
        n112 = Build Array(w30, w29, w28, w27, w26, w25) -> (w24:bool[])
        n113 = Array To Cluster(array=w191) -> (cluster=w192:T1)
        "cluster" <- w192
        n114 = Array To Cluster(array=w24) -> (cluster=w23:T1)
        "cluster 2" <- w23
        n115 = local read "stop"() -> (w266:bool)
        n116 = local write "cluster"(w192) -> ()
        n117 = local write "cluster 2"(w23) -> ()
      }
      n118 = call "IMAQ Create"("Image Name"="AVI", "Image Type"=w14) -> ("New Image"=w12:T3)  [unwired: 3 in, 1 out]
      n119 = call "IMAQ AVI Open"("AVI Path"="AVI Path") -> ("error out"=w19:errorcluster, "Avi Refnum"=w20:T6)  [unwired: 9 in]
      n120 = while {
        tunnel: w20 -> [w287]
        tunnel: w19 -> [w279]
        tunnel: [w286] -> w21
        shift-right: [w281] -> _
        shift-left: "Frame Start" -> [w280]
        tunnel: [w277] -> w15
        tunnel: w12 -> [w276]
        stop <- "stop" stop-if-true
        n121 = call "IMAQ AVI Read Frame"("error in (no error)"=w279, "Frame Number"=w280, "Image"=w276, "Avi Refnum"=w287) -> ("error out"=w277:errorcluster, "Image Out"=→"Image Dst Out":T3, "Avi Refnum (duplicate)"=w286:T6)  [unwired: 4 in, 1 out]
        n122 = Increment(x=w280) -> (x+1=w281:i32)
        n123 = Divide(x=1000.0, y="playtime") -> (x/y=w284:dbl)
        n124 = Wait (ms)(milliseconds to wait=w284) -> ()  [unwired: 1 out]
        "Frame Number" <- w280
      }
      n125 = call "IMAQ AVI Close"("error in (no error)"=w15, "Avi Refnum"=w21) -> ("error out"=w17:errorcluster)  [unwired: 9 in]
      n126 = call <vilib>:"Merge Errors.vi"("error in 3 (no error)"=w10, "error in 2 (no error)"=w11, "error in 1 (no error)"=w17) -> ("error out"=w16:errorcluster)  [unwired: 4 in]
      n127 = call <vilib>:"Clear Errors.vi"("error in (no error)"=w16) -> ()  [unwired: 6 in, 1 out]
    }
  }
  n128 = call-poly "VISA Configure Serial Port"("VISA resource name"="VISA resource name", "Enable Termination\nChar (T)"=FALSE ("Enable Termination\nChar (T)"), "baud rate (9600)"="baud rate (9600)") -> ("VISA resource name out"=w8:refnum<visa-resource-name>, "error out"=w3:errorcluster)  [unwired: 11 in]
  n129 = while {
    shift-right: [w292] -> _
    shift-left: w1 -> [w303]
    tunnel: w8 -> [w302]
    tunnel: [w301] -> w7
    tunnel: w3 -> [w300]
    tunnel: [w299] -> w2
    shift-right: [w291] -> _
    shift-left: w1 -> [w295]
    stop <- w297 stop-if-true
    n130 = local read "cluster 2"() -> (w293:T1)
    n131 = local read "cluster"() -> (w294:T1)
    n132 = Cluster To Array(cluster=w293) -> (array=w298:bool[])
    n133 = Cluster To Array(cluster=w294) -> (array=w296:bool[])
    n134 = Boolean Array To Number(Boolean array=w298) -> (number=w292:u32)
    "number" <- w292
    n135 = Boolean Array To Number(Boolean array=w296) -> (number=w291:u32)
    "number 2" <- w291
    n136 = Equal?(x=w292, y=w303) -> (x = y?=w290:bool)
    n137 = Equal?(x=w291, y=w295) -> (x = y?=w289:bool)
    n138 = Or(x=w290, y=w289) -> (x .or. y?=w288:bool)
    n139 = case shown="False" w288 {
      tunnel: w302 -> [w312 w314]
      tunnel: [w311 w314] -> w301
      tunnel: w292 -> [w310 _]
      tunnel: w300 -> [w309 w313]
      tunnel: [w308 w313] -> w299
      tunnel: w291 -> [w307 _]
      frame #0 {
        n140 = Number To Decimal String(number=w310) -> (decimal integer string=w306:string)  [unwired: 1 in]
        "decimal integer string" <- w306
        n141 = Number To Decimal String(number=w307) -> (decimal integer string=w305:string)  [unwired: 1 in]
        "decimal integer string 2" <- w305
        n142 = Concatenate Strings(w306, w305) -> (w304:string)
        n143 = VISA Write(VISA resource name=w312, write buffer=w304, error in (no error)=w309) -> (VISA resource name out=w311:refnum<visa-resource-name>, error out=w308:errorcluster)  [unwired: 1 out]
      }
      frame #1 {
      }
    }
    n144 = local read "stop"() -> (w297:bool)
  }
  n145 = VISA Close(VISA resource name=w7, error in (no error)=w2) -> ()  [unwired: 1 out]
